vi "Spartan HTTP Busy.vi"(8 "error in (no error)":errorcluster, 11 "HTTP Data":T1 {"object data"."time" format="%0.2f"}) -> (0 "error out":errorcluster)   [LabVIEW 2011]
uses:
  Spartan HTTP Session.ctl
  Addons/internet/http/http_obj.llb/HTTP Session Data.ctl
  Addons/internet/utils/keyedarr.llb/Keyed Array.ctl
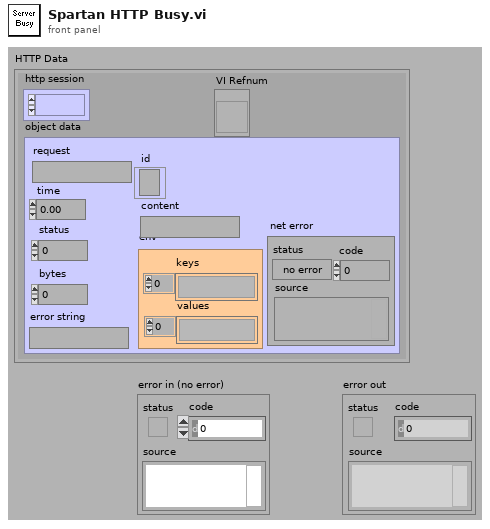
[diagram p1: front panel]
types:
  T1 = typedef "Spartan HTTP Session.ctl" = cluster{"http session":refnum<k1>, "object data":T2, "VI Refnum":refnum<vi>}
  T2 = typedef "HTTP Session Data.ctl" = cluster{"request":string, "time":dbl, "status":i32, "error string":string, "bytes":i32, "env":T3, "content":string, "id":refnum<k5>, "net error":errorcluster}
  T3 = typedef "Keyed Array.ctl" = cluster{"keys":string[], "values":string[]}
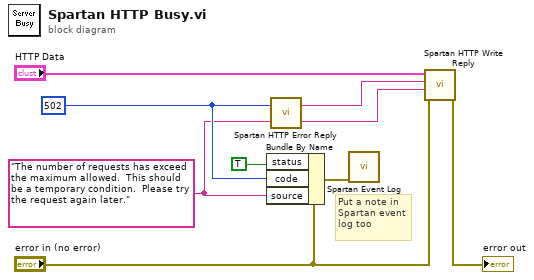
[diagram p0: block diagram]
diagram:
  w6 = "The number of requests has exceed the maximum allowed.  This should be a temporary condition.  Please try the request again later." ("source")
  w7 = 502 ("status code")
  # "Put a note in\nSpartan event\nlog too"
  n1 = Bundle By Name(cluster="error in (no error)", "status"=TRUE, "code"=w7, "source"=w6) -> (w9:errorcluster)
  n2 = call "Spartan HTTP Error Reply.vi"("message"=w6, "status code"=w7) -> ("content"=w3:string, "header"=w4:string)
  n3 = call "Spartan Event Log.vi"("error in (no error)"=w9) -> ()  [unwired: 4 in, 4 out]
  n4 = call "Spartan HTTP Write Reply.vi"("error in (no error)"="error in (no error)", "content"=w3, "header"=w4, "http session"="HTTP Data") -> ("error out"=→"error out":errorcluster)  [unwired: 7 out]
